vi "Configure Marker State.vi"(7 "Marker On":bool, 8 "error in (no error)":errorcluster, 10 "Marker Number":u8=1, 11 "VNA-Ag87xx in":refnum<class "VNA-Ag87xx.lvclass">) -> (0 "error out":errorcluster, 3 "VNA-Ag87xx out":refnum<class "VNA-Ag87xx.lvclass">)   [LabVIEW 2020, in "VNA-Ag87xx.lvclass"]
doc: "Configure the marker state.\nThe marker is on the active trace."
uses:
  VNA-Ag87xx.lvclass
  C:/Sandbox/RF Bench/Source Code/WiSpry Test Framework/Instruments/Instrument.lvclass
  Instrument.lvclass
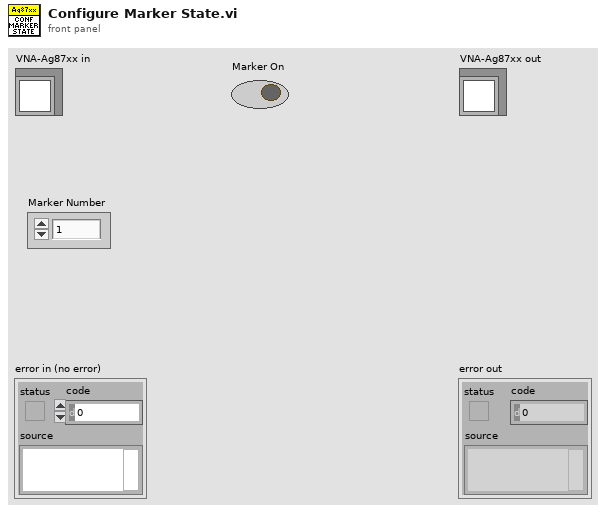
[diagram p1: front panel]
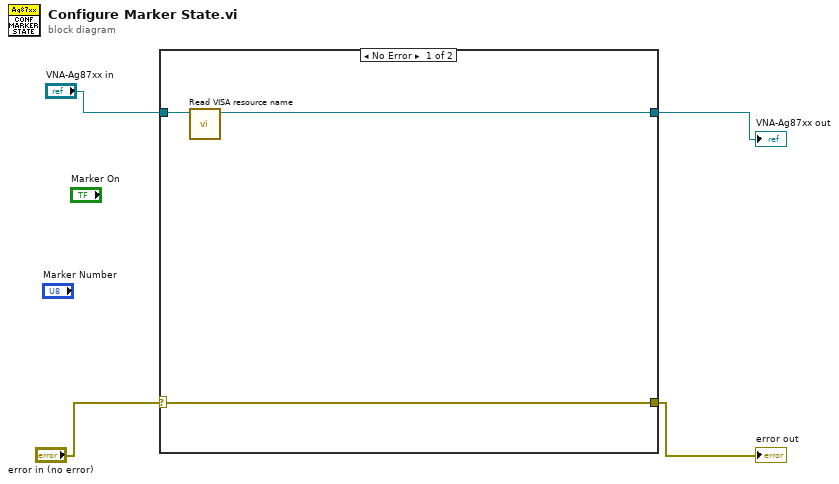
[diagram p0: block diagram]
diagram:
  n1 = case shown="No Error" "error in (no error)" {
    selector: "error in (no error)" -> [w5 w8]
    tunnel: [w6 w9] -> w3
    tunnel: "VNA-Ag87xx in" -> [w7 w9]
    tunnel: [w5 w8] -> w4
    frame No Error {
      n2 = call "Read VISA resource name.vi"("Instrument in"=w7) -> ("Instrument out"=w6:refnum<class "VNA-Ag87xx.lvclass">)  [unwired: 9 in, 1 out]
    }
    frame Error {
    }
  }
  "error out" <- w4
  "VNA-Ag87xx out" <- w3
